vi "Framework_Initialize.vi"(8 "error in (no error)":errorcluster, 11 "AB_EXE in":refnum<class "AB_EXE.lvclass">) -> (0 "error out":errorcluster, 1 "helpTopics":string[](array[string]), 2 "pageTitles":string[](array[string]), 3 "AB_EXE out":refnum<class "AB_EXE.lvclass">, 4 "helpFile":string, 5 "pages":path[](array[path]))   [LabVIEW 2020, in "AB_EXE.lvclass"]
uses:
  <vilib>/AppBuilder/AB_Classes/EXE/AB_EXE.lvclass
panel:
  in  "pageTitles_EXE":string[](array[string])=["Information", "Source Files", "Destinations", "Source File Settings", "Icon", "Advanced", "Additional Exclusions", "Version Information", "Windows Security", "Shared Variable Deployment", "Run-Time Languages", "Web Services", "Pre/Post Build Actions", "Preview"]
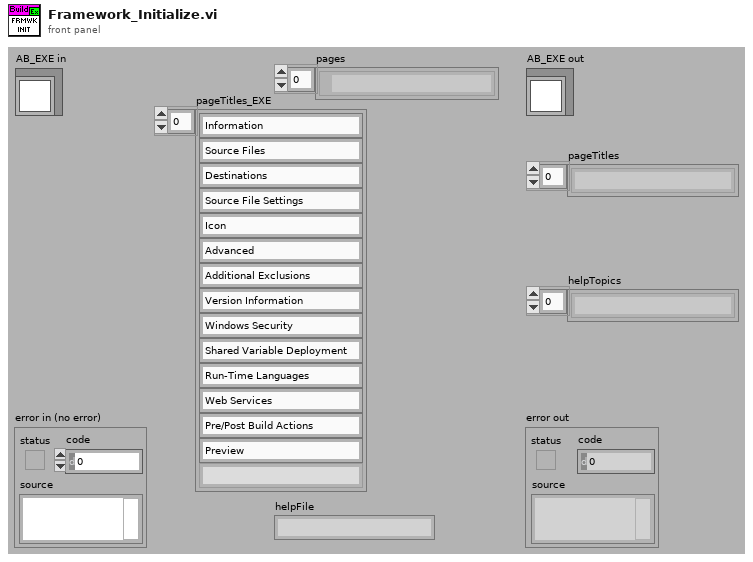
[diagram p1: front panel]
types:
  T1 = enum32{"invalid OS target", "Mac OS", "Windows 3.1", "Windows 95/NT", "Solaris 1", "Solaris 2", "HP-UX", "PowerMAX", "Linux", "Irix", "Rhapsody", "BeOS", "AIX", "OSF1", "VxWorks", "PharLap", "Carbon", "RTX", "Windows x64", "Linux x64", "Mac OS X x64"}
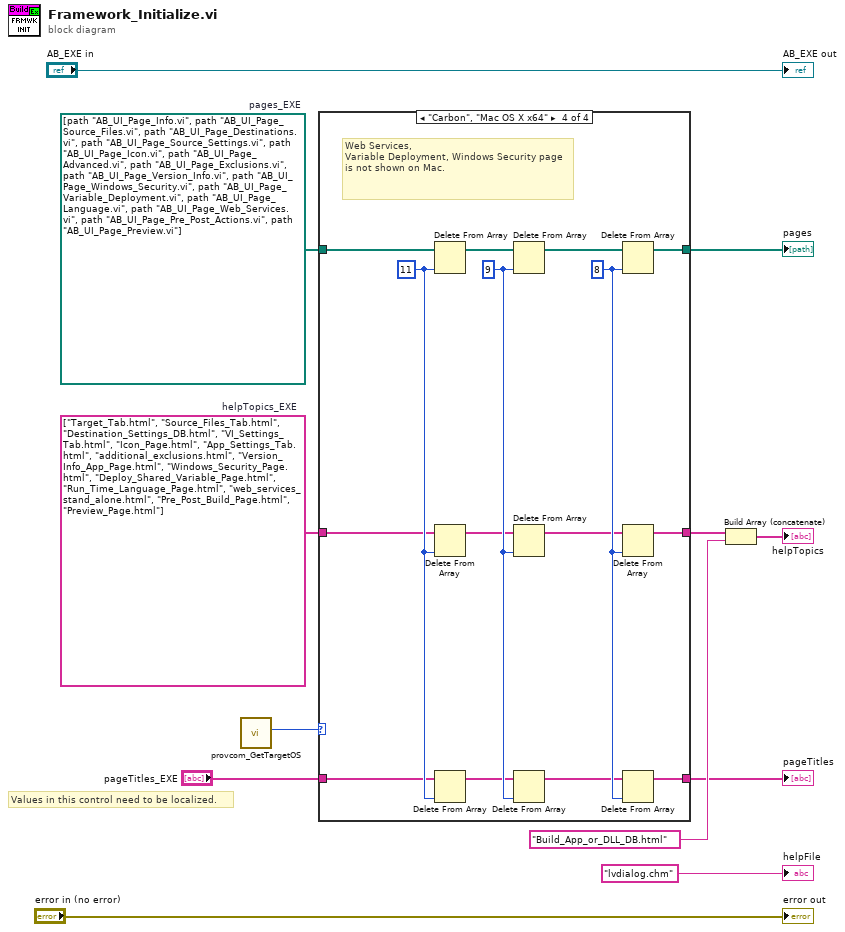
[diagram p0: block diagram]
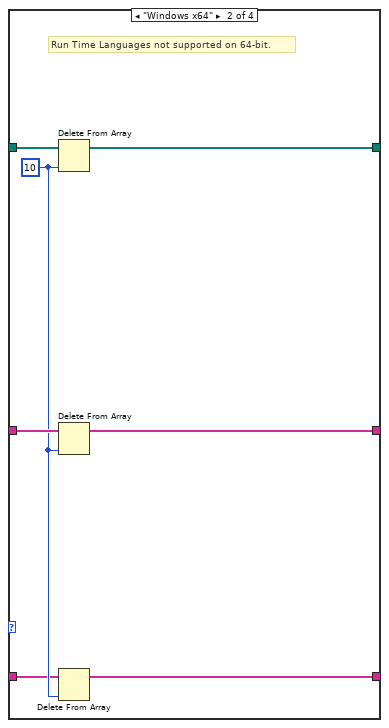
[diagram p3: hidden frame]
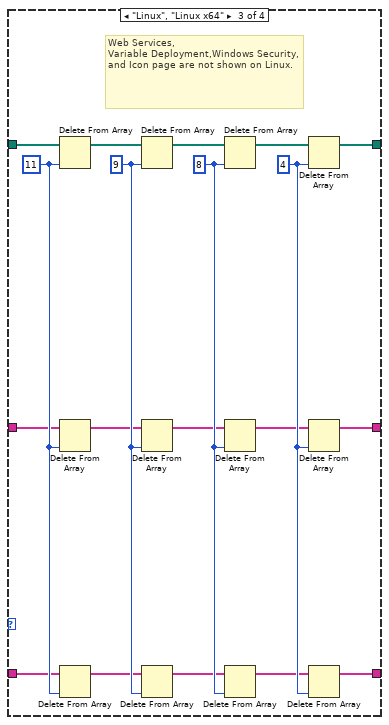
[diagram p4: hidden frame]
diagram:
  w1 = string[] ["Target_Tab.html", "Source_Files_Tab.html", "Destination_Settings_DB.html", "VI_Settings_Tab.html", "Icon_Page.html", "App_Settings_Tab.html", "additional_exclusions.html", "Version_Info_App_Page.html", "Windows_Security_Page.html", "Deploy_Shared_Variable_Page.html", "Run_Time_Language_Page.html", "web_services_stand_alone.html", "Pre_Post_Build_Page.html", "Preview_Page.html"]  # helpTopics_EXE
  w2 = path[] [path "AB_UI_Page_Info.vi", path "AB_UI_Page_Source_Files.vi", path "AB_UI_Page_Destinations.vi", path "AB_UI_Page_Source_Settings.vi", path "AB_UI_Page_Icon.vi", path "AB_UI_Page_Advanced.vi", path "AB_UI_Page_Exclusions.vi", path "AB_UI_Page_Version_Info.vi", path "AB_UI_Page_Windows_Security.vi", path "AB_UI_Page_Variable_Deployment.vi", path "AB_UI_Page_Language.vi", path "AB_UI_Page_Web_Services.vi", path "AB_UI_Page_Pre_Post_Actions.vi", path "AB_UI_Page_Preview.vi"]  # pages_EXE
  # "11"
  # "10"
  # "8"
  # "9"
  # "4"
  # "7"
  # "Values in this control need to be localized."
  n1 = call <resource>:"provcom_GetTargetOS.vi"() -> ("App.TargetOS"=w9:T1)  [unwired: 11 out]
  n2 = case shown="\"Carbon\", \"Mac OS X x64\"" w9 {
    tunnel: [w14 w16 w40 w53] -> w8
    tunnel: [w13 w17 w39 w51] -> w5
    tunnel: "pageTitles_EXE" -> [w15 w19 w24 w43]
    tunnel: [w15 w18 w41 w49] -> w3
    tunnel: w2 -> [w14 w22 w28 w47]
    tunnel: w1 -> [w13 w21 w26 w45]
    frame Default {
    }
    frame "Windows x64" {
      w20 = 10 ("index")
      # "Run Time Languages not supported on 64-bit."
      n3 = Delete From Array(array=w22, index=w20) -> (array with subset deleted=w16:path[])  [unwired: 1 in, 1 out]
      n4 = Delete From Array(array=w21, index=w20) -> (array with subset deleted=w17:string[])  [unwired: 1 in, 1 out]
      n5 = Delete From Array(array=w19, index=w20) -> (array with subset deleted=w18:string[])  [unwired: 1 in, 1 out]
    }
    frame "Linux", "Linux x64" {
      w29 = 11 ("index")
      w36 = 8 ("index")
      w37 = 9 ("index")
      w38 = 4 ("index")
      # "Web Services,\nVariable Deployment,Windows Security, and Icon page are not shown on Linux."
      n6 = Delete From Array(array=w28, index=w29) -> (array with subset deleted=w27:path[])  [unwired: 1 in, 1 out]
      n7 = Delete From Array(array=w26, index=w29) -> (array with subset deleted=w25:string[])  [unwired: 1 in, 1 out]
      n8 = Delete From Array(array=w24, index=w29) -> (array with subset deleted=w23:string[])  [unwired: 1 in, 1 out]
      n9 = Delete From Array(array=w27, index=w37) -> (array with subset deleted=w35:path[])  [unwired: 1 in, 1 out]
      n10 = Delete From Array(array=w25, index=w37) -> (array with subset deleted=w34:string[])  [unwired: 1 in, 1 out]
      n11 = Delete From Array(array=w23, index=w37) -> (array with subset deleted=w33:string[])  [unwired: 1 in, 1 out]
      n12 = Delete From Array(array=w35, index=w36) -> (array with subset deleted=w30:path[])  [unwired: 1 in, 1 out]
      n13 = Delete From Array(array=w34, index=w36) -> (array with subset deleted=w31:string[])  [unwired: 1 in, 1 out]
      n14 = Delete From Array(array=w33, index=w36) -> (array with subset deleted=w32:string[])  [unwired: 1 in, 1 out]
      n15 = Delete From Array(array=w30, index=w38) -> (array with subset deleted=w40:path[])  [unwired: 1 in, 1 out]
      n16 = Delete From Array(array=w31, index=w38) -> (array with subset deleted=w39:string[])  [unwired: 1 in, 1 out]
      n17 = Delete From Array(array=w32, index=w38) -> (array with subset deleted=w41:string[])  [unwired: 1 in, 1 out]
    }
    frame "Carbon", "Mac OS X x64" {
      w48 = 11 ("index")
      w55 = 8 ("index")
      w56 = 9 ("index")
      # "Web Services,\nVariable Deployment, Windows Security page is not shown on Mac."
      n18 = Delete From Array(array=w47, index=w48) -> (array with subset deleted=w46:path[])  [unwired: 1 in, 1 out]
      n19 = Delete From Array(array=w45, index=w48) -> (array with subset deleted=w44:string[])  [unwired: 1 in, 1 out]
      n20 = Delete From Array(array=w43, index=w48) -> (array with subset deleted=w42:string[])  [unwired: 1 in, 1 out]
      n21 = Delete From Array(array=w46, index=w56) -> (array with subset deleted=w54:path[])  [unwired: 1 in, 1 out]
      n22 = Delete From Array(array=w44, index=w56) -> (array with subset deleted=w52:string[])  [unwired: 1 in, 1 out]
      n23 = Delete From Array(array=w42, index=w56) -> (array with subset deleted=w50:string[])  [unwired: 1 in, 1 out]
      n24 = Delete From Array(array=w54, index=w55) -> (array with subset deleted=w53:path[])  [unwired: 1 in, 1 out]
      n25 = Delete From Array(array=w52, index=w55) -> (array with subset deleted=w51:string[])  [unwired: 1 in, 1 out]
      n26 = Delete From Array(array=w50, index=w55) -> (array with subset deleted=w49:string[])  [unwired: 1 in, 1 out]
    }
  }
  "pages" <- w8
  "pageTitles" <- w3
  n27 = Build Array (concatenate)(w5, "Build_App_or_DLL_DB.html" ("HTML filename")) -> (→"helpTopics":string[])
  "error out" <- "error in (no error)"
  "AB_EXE out" <- "AB_EXE in"
  "helpFile" <- "lvdialog.chm" ("CHM or HLP filename (lvdialog.chm)")
